vi "ClusterwitharrayI8.vi"(1 "Cluster In":cluster{"Array In":i8[], "Numeric Input":i8}, 2 "Base":i8) -> (0 "Cluster Out":cluster{"Array Out":i8[], "Numeric Output":i8})   [LabVIEW 2010]
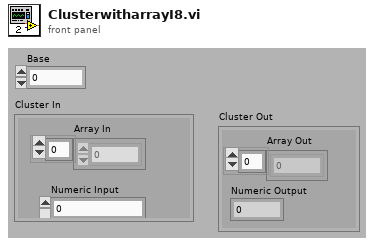
[diagram p1: front panel]
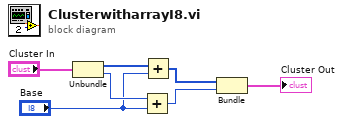
[diagram p0: block diagram]
diagram:
  n1 = Unbundle("Cluster In") -> ("Array In"=w7:i8[], "Numeric Input"=w6:i8)
  n2 = Add(x=w6, y="Base") -> (x+y=w4:i8)
  n3 = Add(x=w7, y="Base") -> (x+y=w5:i8[])
  n4 = Bundle(w5, w4) -> (→"Cluster Out":cluster{i8[], i8})  [unwired: 1 out]
